vi "TAT-Stop.vi"(7 "Enum":enum16{"Read", "Write"}(ring)=enum."Write", 11 "Stop":bool) -> (3 "Stop":bool)   [LabVIEW 2017]
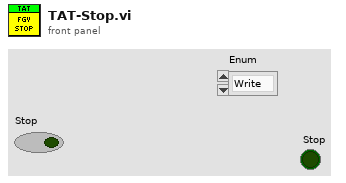
[diagram p1: front panel]
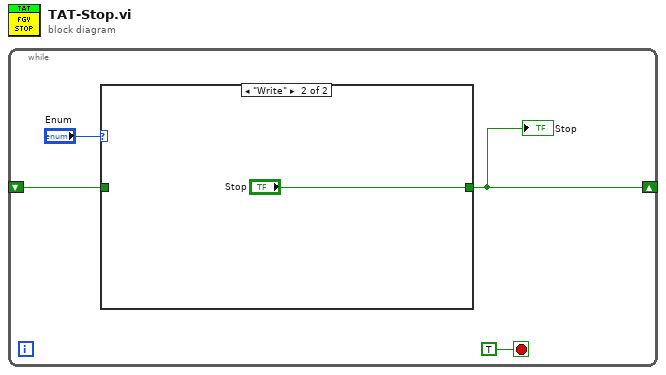
[diagram p0: block diagram]
diagram:
  n1 = while {
    shift-right: [w1] -> _
    shift-left: _ -> [w2]
    stop <- TRUE stop-if-true
    n2 = case shown="\"Write\"" "Enum" {
      tunnel: [w5 "Stop"] -> w1
      tunnel: w2 -> [w5 _]
      frame "Read", Default {
      }
      frame "Write" {
      }
    }
    "Stop" <- w1
  }
